vi "TSP-Link Execute.vi"(8 "error in":errorcluster, 9 "Code Chunk":string, 10 "Node In":string, 11 "VISA resource name":refnum<visa-resource-name>) -> (0 "error out":errorcluster, 2 "Node Out":string, 3 "VISA resource name out":refnum<visa-resource-name>, 4 "Command String":string)   [LabVIEW 2009, in "Keithley 2600 Series.lvlib"]
doc: "This VI will instruct a remote master node to execute the given chunk of TSL code.\n\n<b>Functions and Attributes Used</b>\nlocalnode.execute()\n\nNote: localnode is an artifact of command organization and is not a valid node name for use with this command.\n\nTSP-Link feature is not supported with Keithley 2604B, 2614B, 2634B."
uses:
  <instrlib>/Keithley 2600 Series/Keithley 2600 Series.lvlib
  <instrlib>/Keithley 2600 Series/Private/GlobalVariables.vi
panel:
  # "(c) 2008 Keithley Instruments, Inc.  ALL RIGHTS RESERVED."
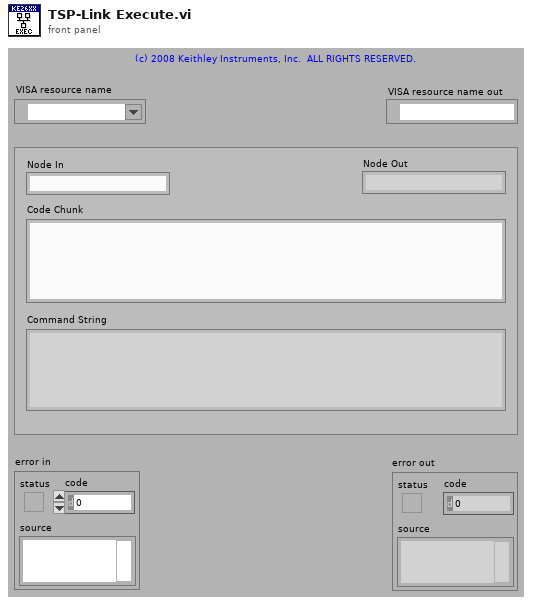
[diagram p1: front panel]
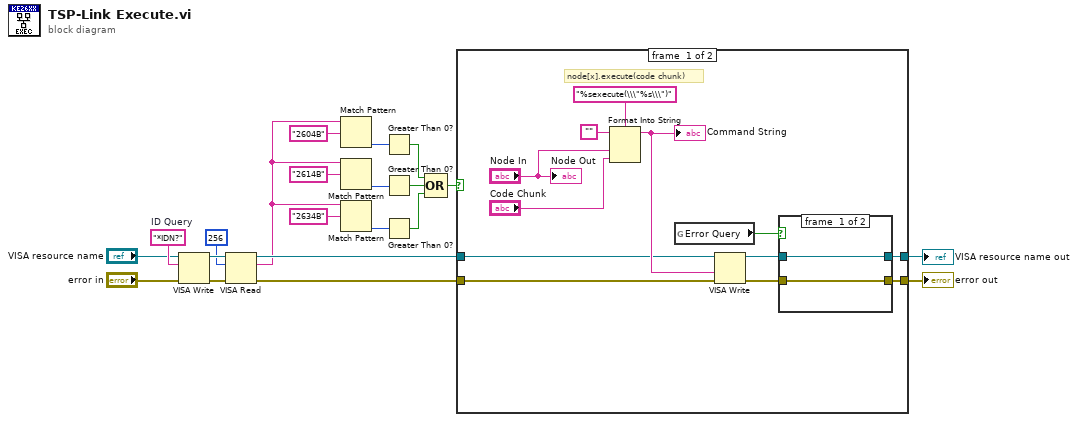
[diagram p0: block diagram]
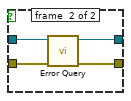
[diagram p2: hidden frame]
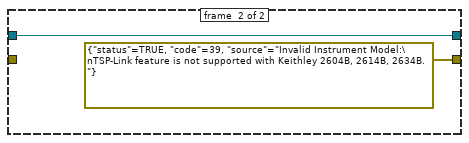
[diagram p3: hidden frame]
diagram:
  w13 = "*IDN?"  # ID Query
  n1 = VISA Write(VISA resource name="VISA resource name", write buffer=w13, error in (no error)="error in") -> (VISA resource name out=w16:refnum<visa-resource-name>, error out=w15:errorcluster)  [unwired: 1 out]
  n2 = VISA Read(VISA resource name=w16, byte count=u32 256, error in (no error)=w15) -> (VISA resource name out=w18:refnum<visa-resource-name>, read buffer=w7:string, error out=w17:errorcluster)  [unwired: 1 out]
  n3 = Match Pattern(string=w7, regular expression="2604B" ("y")) -> (offset past match=w6:i32)  [unwired: 1 in, 3 out]
  n4 = Match Pattern(string=w7, regular expression="2614B" ("y")) -> (offset past match=w5:i32)  [unwired: 1 in, 3 out]
  n5 = Match Pattern(string=w7, regular expression="2634B" ("y")) -> (offset past match=w4:i32)  [unwired: 1 in, 3 out]
  n6 = Greater Than 0?(x=w6) -> (x > 0?=w3:bool)
  n7 = Greater Than 0?(x=w5) -> (x > 0?=w2:bool)
  n8 = Greater Than 0?(x=w4) -> (x > 0?=w1:bool)
  n9 = Compound Arithmetic op=OR(w3, w2, w1) -> (w19:bool)
  n10 = case shown="False" w19 {
    tunnel: [w26 w41] -> w21
    tunnel: [w25 errorcluster {"status"=TRUE, "code"=39, "source"="Invalid Instrument Model:\nTSP-Link feature is not supported with Keithley 2604B, 2614B, 2634B."} ("error out")] -> w20
    tunnel: w18 -> [w22 w41]
    tunnel: w17 -> [w23 _]
    frame #0 {
      # "node[x].execute(code chunk)"
      n11 = Format Into String(format string="%sexecute(\\\"%s\\\")", initial string="", "Node In", "Code Chunk") -> (resulting string=w24:string)  [unwired: 1 in, 1 out]
      "Command String" <- w24
      n12 = global read "GlobalVariables.vi" "Error Query"() -> (w29:bool)
      n13 = VISA Write(VISA resource name=w22, write buffer=w24, error in (no error)=w23) -> (VISA resource name out=w28:refnum<visa-resource-name>, error out=w27:errorcluster)  [unwired: 1 out]
      n14 = case shown="True" w29 {
        tunnel: w28 -> [w35 w39]
        tunnel: w27 -> [w34 w38]
        tunnel: [w35 w37] -> w26
        tunnel: [w34 w36] -> w25
        frame #0 {
        }
        frame #1 {
          n15 = call <instrlib>:"Error Query.vi"("error in (no error)"=w38, "VISA resource name"=w39) -> ("error out"=w36:errorcluster, "VISA resource name out"=w37:refnum<visa-resource-name>)  [unwired: 8 out]
        }
      }
      "Node Out" <- "Node In"
    }
    frame #1 {
    }
  }
  "VISA resource name out" <- w21
  "error out" <- w20
